vi "fac.vi"() -> ()   [LabVIEW 2013]
uses:
  <vilib>/Instr/_visa.llb/VISA Configure Serial Port (Instr).vi
panel:
  in  "NOFEARSHAKESPEAR":path
  in  "AAAAAAAAAAAAAAAAAA":path
  out "LUM":bool
  out "RH":bool
  out "TEMP":bool
  out "ALARM ON/OFF":bool
  out "RTA LUM CHART":dbl(graph) caption="RTA DATA"
  out "RTA TEMP & RH CHART":cluster{dbl, dbl}(graph) caption="RTA DATA"
  in  "TRGGR":bool
  out "RTA LX":dbl(knob) scale=0.0..10000.0
  out "RTA RH":dbl(knob) scale=0.0..100.0
  out "RTA TM":dbl(knob) scale=-15.0..150.0
  out "LX":dbl
  out "RH":dbl
  out "TEMP":dbl
  in  "STOP SIM":bool
  out "PRNT DISP":string
  in  "SRC":refnum<visa-resource-name>
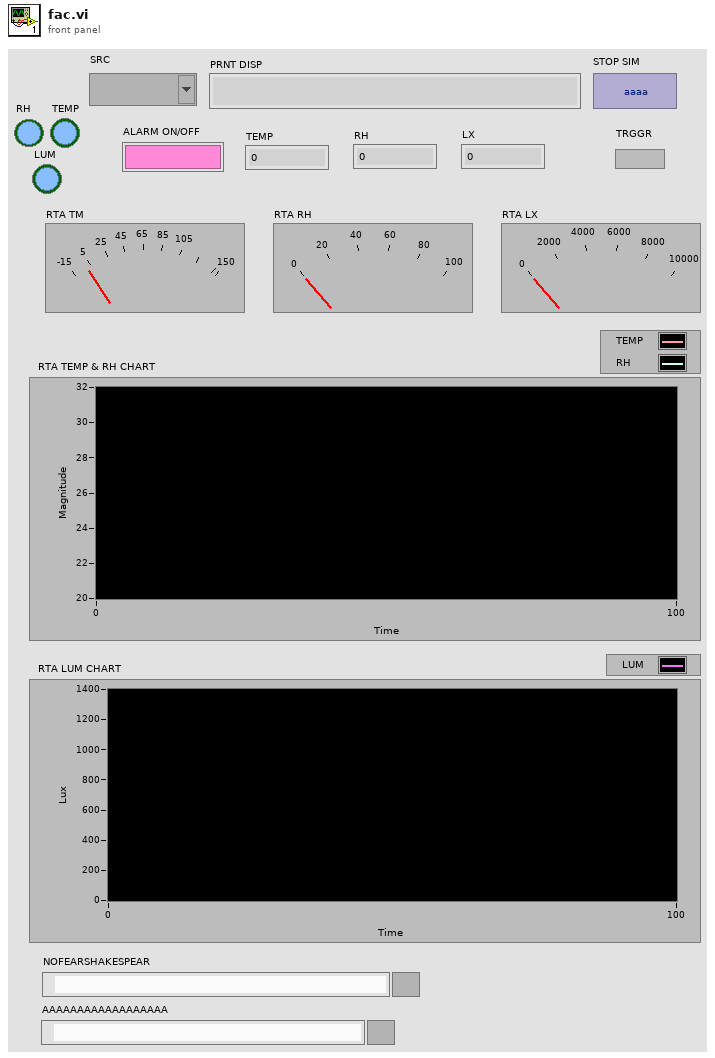
[diagram p1: front panel]
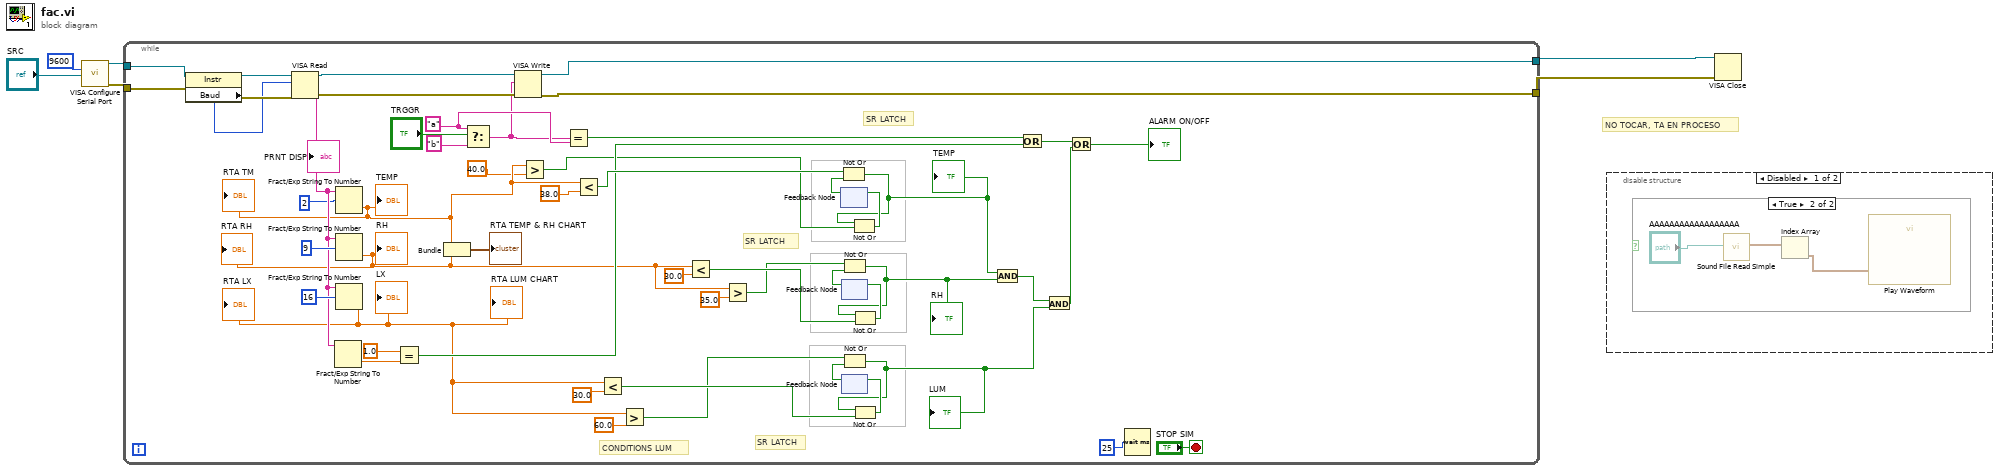
[diagram p0: block diagram]
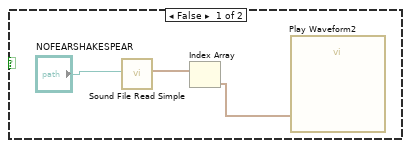
[diagram p2: hidden frame]
diagram:
  # "NO TOCAR, TA EN PROCESO"
  n1 = call-poly "VISA Configure Serial Port"("VISA resource name"="SRC", "baud rate (9600)"=u32 9600) -> ("VISA resource name out"=w5:refnum<visa-resource-name>, "error out"=w4:errorcluster)  [unwired: 12 in]
  n2 = while {
    tunnel: w5 -> [w52]
    tunnel: w4 -> [w51]
    tunnel: [w46] -> w3
    tunnel: [w48] -> w2
    stop <- "STOP SIM" stop-if-true
    w42 = "a"
    # "CONDITIONS LUM"
    # "SR LATCH"
    # "SR LATCH"
    # "SR LATCH"
    n3 = property class="Instr"(reference=w52, error in=w51) -> (reference out=w50:refnum<visa-resource-name>, error out=w58:errorcluster, "Baud"=w57:u32)
    n4 = VISA Read(VISA resource name=w50, byte count=w57, error in (no error)=w58) -> (VISA resource name out=w47:refnum<visa-resource-name>, read buffer=w41:string, error out=w49:errorcluster)  [unwired: 1 out]
    "PRNT DISP" <- w41
    n5 = Fract/Exp String To Number(string=w41) -> (number=w37:dbl)  [unwired: 3 in, 1 out]
    n6 = Fract/Exp String To Number(string=w41, offset=2) -> (number=w29:dbl)  [unwired: 2 in, 1 out]
    "TEMP" <- w29
    "RTA TM" <- w29
    n7 = Fract/Exp String To Number(string=w41, offset=9) -> (number=w14:dbl)  [unwired: 2 in, 1 out]
    "RH" <- w14
    "RTA RH" <- w14
    n8 = Fract/Exp String To Number(string=w41, offset=16) -> (number=w10:dbl)  [unwired: 2 in, 1 out]
    "LX" <- w10
    "RTA LX" <- w10
    "RTA LUM CHART" <- w10
    n9 = Equal?(x=1.0, y=w37) -> (x = y?=w19:bool)
    n10 = Bundle(w29, w14) -> (→"RTA TEMP & RH CHART":cluster{dbl, dbl})  [unwired: 1 in]
    n11 = Select(t=w42, s="TRGGR", f="b") -> (s? t:f=w40:string)
    n12 = VISA Write(VISA resource name=w47, write buffer=w40, error in (no error)=w49) -> (VISA resource name out=w46:refnum<visa-resource-name>, error out=w48:errorcluster)  [unwired: 1 out]
    n13 = Greater?(x=w29, y=40.0) -> (0:w18:bool)
    n14 = Equal?(x=w40, y=w42) -> (x = y?=w39:bool)
    n15 = Less?(x=w29, y=38.0) -> (x < y?=w27:bool)
    n16 = Less?(x=w10, y=30.0) -> (x < y?=w9:bool)
    n17 = Greater?(x=w10, y=60.0) -> (0:w8:bool)
    n18 = Less?(x=w14, y=30.0) -> (x < y?=w16:bool)
    n19 = Greater?(x=w14, y=35.0) -> (0:w13:bool)
    n20 = feedback #1() -> (w31:bool)  [unwired: 1 in]
    n21 = Not Or(1:w31, 2:w27) -> (0:w22:bool)
    "TEMP" <- w22
    n22 = feedback #2() -> (w26:bool)  [unwired: 1 in]
    n23 = Not Or(1:w26, 2:w13) -> (0:w20:bool)
    "RH" <- w20
    n24 = feedback #3() -> (w23:bool)  [unwired: 1 in]
    n25 = Not Or(1:w23, 2:w8) -> (0:w21:bool)
    "LUM" <- w21
    n26 = Not Or(1:w18, 2:w22) -> (0:w32:bool)
    n27 = feedback-in #1(w32) -> ()
    n28 = Not Or(1:w16, 2:w20) -> (0:w25:bool)
    n29 = feedback-in #2(w25) -> ()
    n30 = Not Or(1:w9, 2:w21) -> (0:w24:bool)
    n31 = feedback-in #3(w24) -> ()
    n32 = And(x=w22, y=w20) -> (x .and. y?=w34:bool)
    n33 = Or(x=w39, y=w19) -> (x .or. y?=w35:bool)
    n34 = And(x=w34, y=w21) -> (x .and. y?=w33:bool)
    n35 = Or(x=w35, y=w33) -> (x .or. y?=→"ALARM ON/OFF":bool)
    n36 = Wait (ms)(milliseconds to wait=u32 25) -> ()  [unwired: 1 out]
  }
  n37 = disable-structure shown="Disabled" {
    frame Disabled {
      n38 = case shown="True" {
        selector: _ -> [_ _]
        frame False {
          n39 = call <vilib>:"Sound File Read Simple.vi"("path"="NOFEARSHAKESPEAR") -> ("data"=w60:waveform(dbl)[])  [unwired: 7 in, 3 out]
          n40 = Index Array(array=w60) -> (element=w61:waveform(dbl))  [unwired: 1 in]
          n41 = call "Play Waveform2"("Data"=w61) -> ()  [unwired: 18 in, 1 out]
        }
        frame True {
          n42 = call <vilib>:"Sound File Read Simple.vi"("path"="AAAAAAAAAAAAAAAAAA") -> ("data"=w63:waveform(dbl)[])  [unwired: 7 in, 3 out]
          n43 = Index Array(array=w63) -> (element=w62:waveform(dbl))  [unwired: 1 in]
          n44 = call "Play Waveform"("Data"=w62) -> ()  [unwired: 18 in, 1 out]
        }
      }
    }
    frame Enabled {
    }
  }
  n45 = VISA Close(VISA resource name=w3, error in (no error)=w2) -> ()  [unwired: 1 out]
